vi "OSC_picture.vi"(6 "Falling(T)/Rising(F)":bool, 7 "trig level":dbl format="%#_13g", 8 "error in (no error)":errorcluster, 9 "channels":string="0", 10 "timeout (s) 2":dbl caption="Timeout(s)" format="%.2f", 11 "instrument handle":refnum<k15>) -> (0 "error out":errorcluster, 1 "Waveform Graph":waveform(dbl)[](graph), 2 "the value of the waveform":dbl format="%0.2f", 3 "instrument handle out":refnum<k15>)   [LabVIEW 2013]
uses:
  <instrlib>/niScope/Controls/niScope timestamp type.ctl
  <vilib>/Analysis/baseanly.llb/Mean (DBL).vi
  <vilib>/measure/mamon.llb/Trigger Detection for 1 Channel (obs).vi
  <vilib>/Analysis/NI_AALBase.lvlib
  <vilib>/measure/NI_MAPro.lvlib
panel:
  out "output waveform":waveform(dbl)={"t0"=timestamp(-2.500000000349445e-07 s since 1904-01-01), "dt"=1e-09, "Y"=array[2494 elements]}
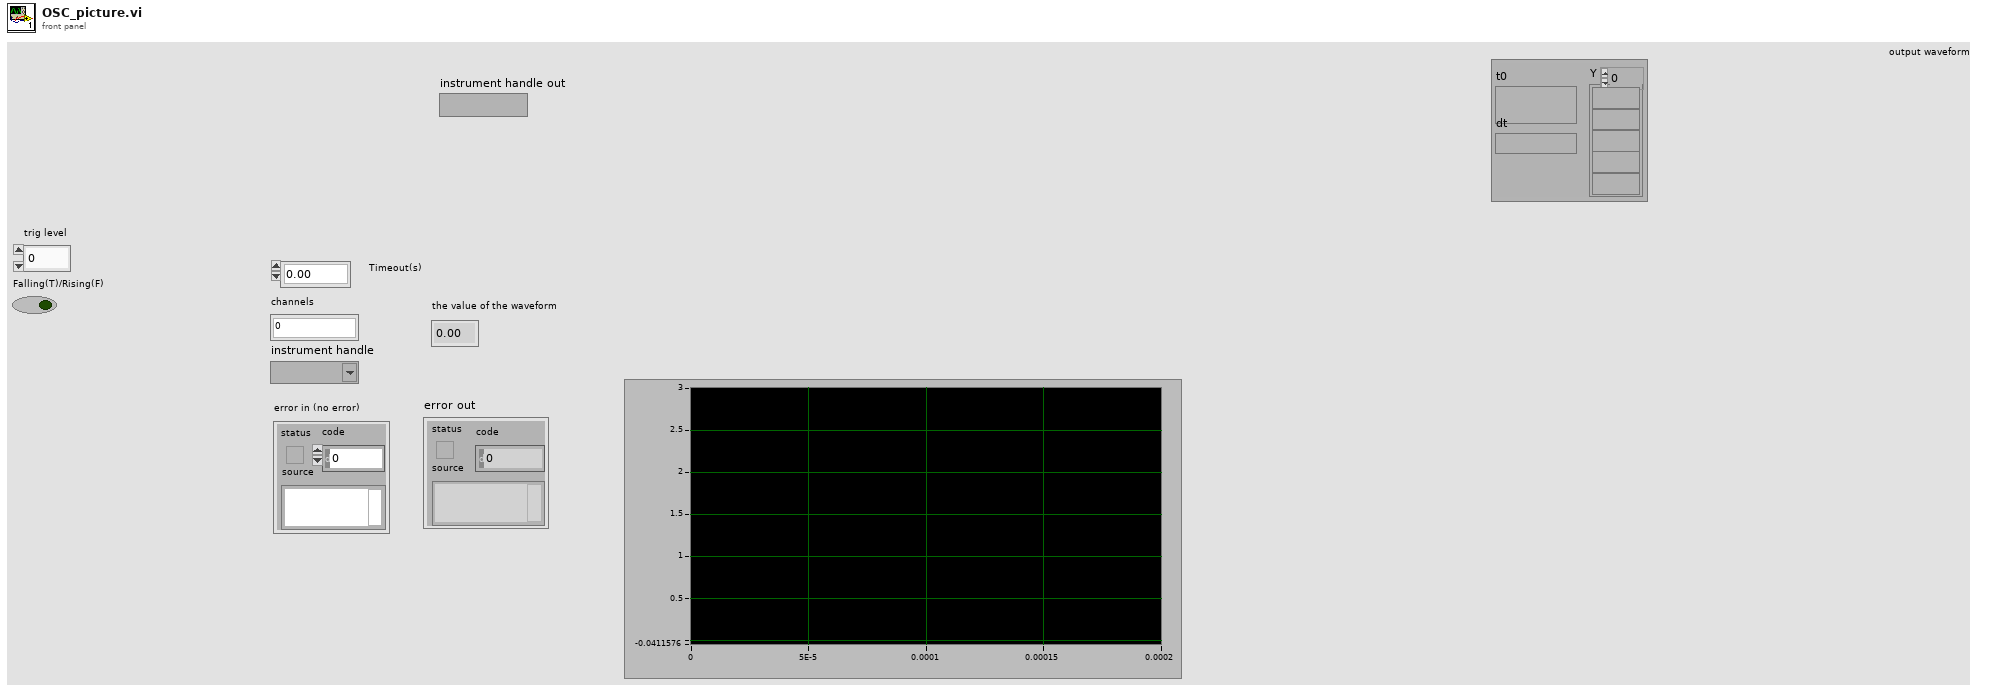
[diagram p1: front panel]
types:
  T1 = typedef "niScope timestamp type.ctl" = i32
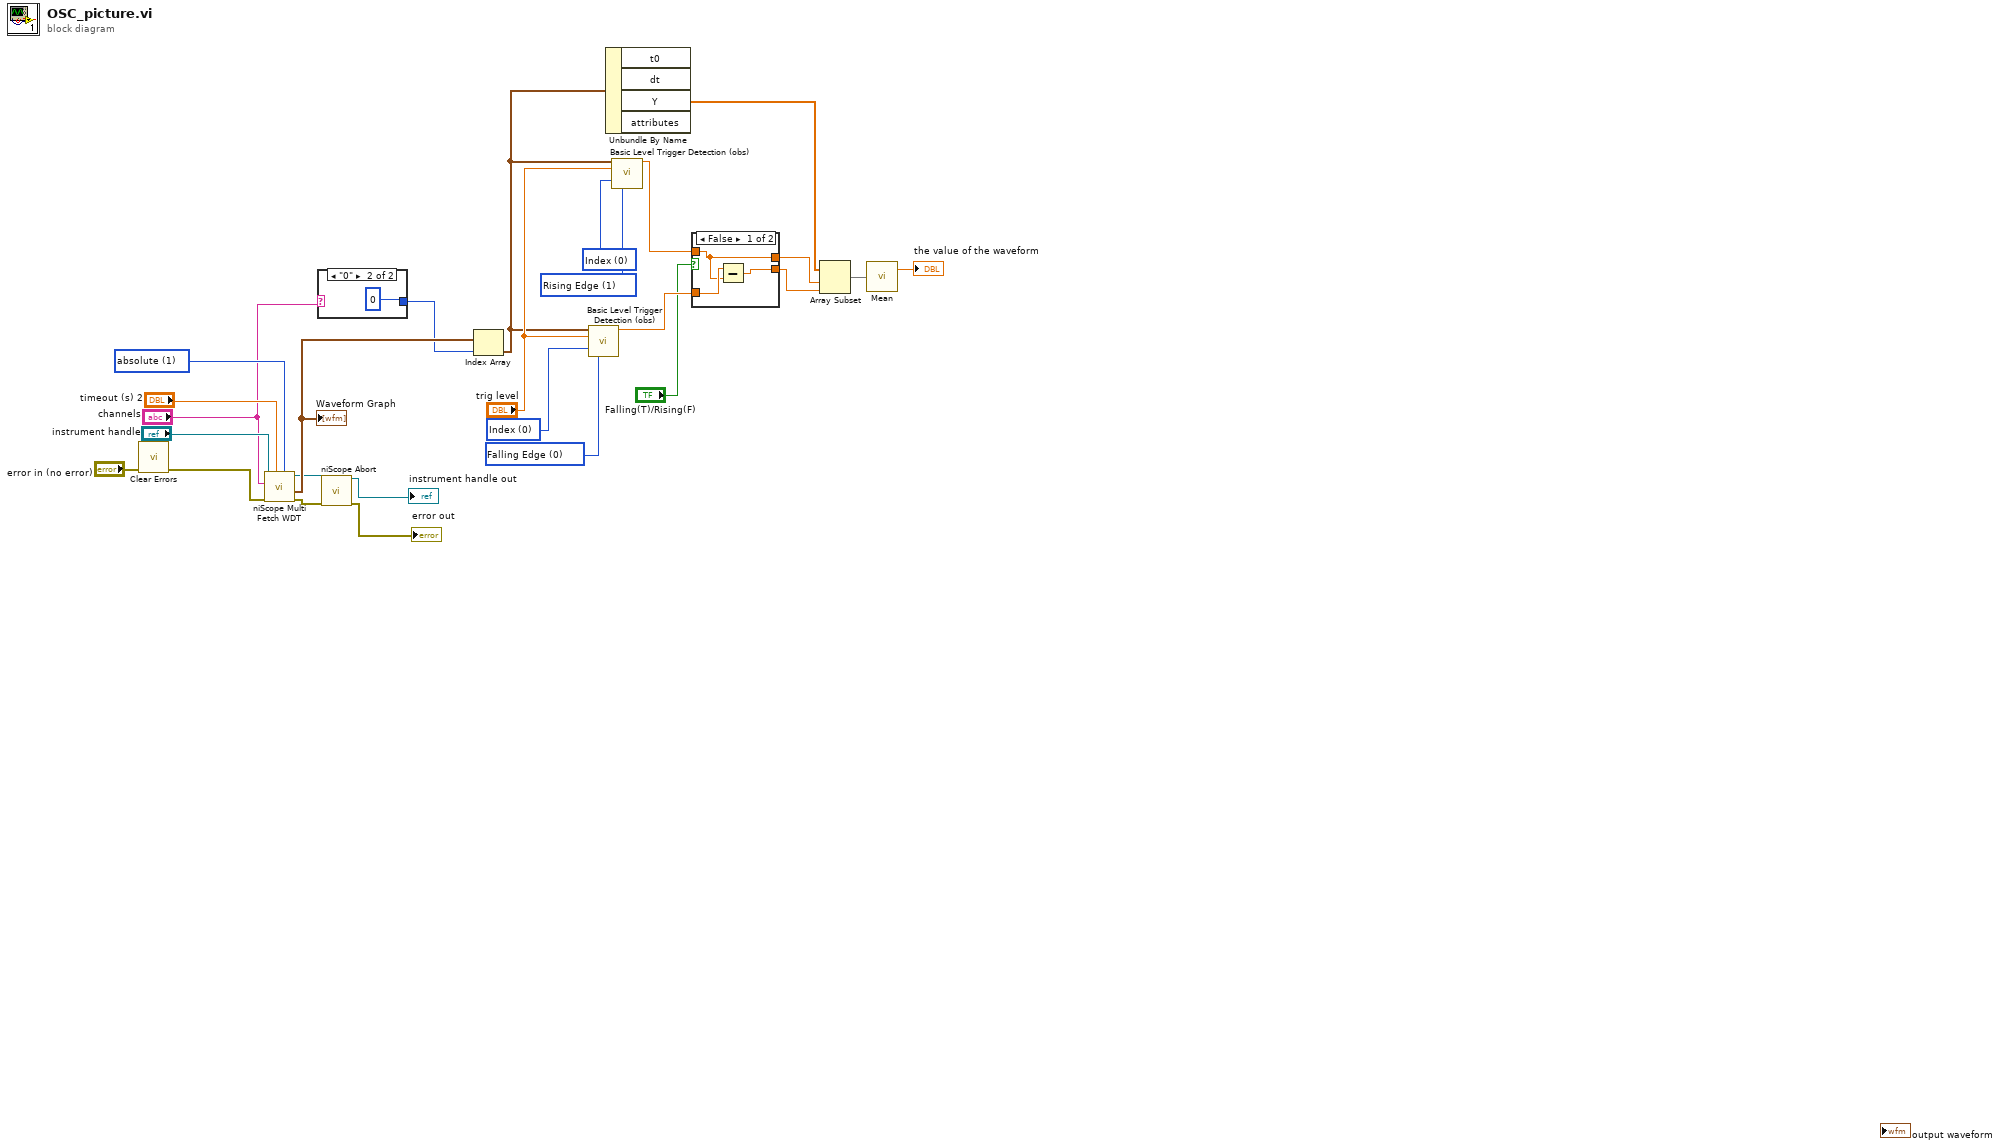
[diagram p0: block diagram]
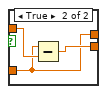
[diagram p2: hidden frame]
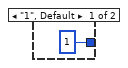
[diagram p3: hidden frame]
diagram:
  w14 = u16 0 items=["Index", "Time"] ("location mode")
  w15 = u16 1 items=["Falling Edge", "Rising Edge"] ("trigger slope")
  w17 = u16 0 items=["Index", "Time"] ("location mode")
  w16 = u16 0 items=["Falling Edge", "Rising Edge"] ("trigger slope")
  w25 = T1 1 items=["relative", "absolute"] ("timestamp Type")
  n1 = call <vilib>:"Clear Errors.vi"("error in (no error)"="error in (no error)") -> ("error out"=w22:errorcluster)  [unwired: 6 in]
  n2 = call "niScope Multi Fetch WDT.vi"("timestamp Type"=w25, "timeout"="timeout (s) 2", "error in"=w22, "channels"="channels", "instrument handle"="instrument handle") -> ("error out"=w3:errorcluster, "wfm"=w21:waveform(dbl)[], "instrument handle out"=w4:refnum<k15>)  [unwired: 3 in, 1 out]
  "Waveform Graph" <- w21
  n3 = case shown="\"0\"" "channels" {
    tunnel: [1 ("index") 0 ("index")] -> w20
    frame "1", Default {
    }
    frame "0" {
    }
  }
  n4 = call <instrlib>:"niScope Abort.vi"("instrument handle"=w4, "error in"=w3) -> ("instrument handle out"=→"instrument handle out":refnum<k15>, "error out"=→"error out":errorcluster)  [unwired: 12 in]
  n5 = Index Array(array=w21, index=w20) -> (element=w10:waveform(dbl))
  n6 = call-poly <vilib>:"Basic Level Trigger Detection (obs).vi"("signal in"=w10, "level"="trig level", "location mode"=w17, "trigger slope"=w16) -> ("trigger location"=w12:dbl)  [unwired: 9 in, 2 out]
  n7 = Unbundle By Name(w10) -> ("Y"=w9:dbl[])  [unwired: 3 out]
  n8 = call-poly <vilib>:"Basic Level Trigger Detection (obs).vi"("signal in"=w10, "level"="trig level", "location mode"=w14, "trigger slope"=w15) -> ("trigger location"=w11:dbl)  [unwired: 9 in, 2 out]
  n9 = case shown="False" "Falling(T)/Rising(F)" {
    tunnel: w12 -> [w30 w32]
    tunnel: w11 -> [w29 w34]
    tunnel: [w31 w33] -> w8
    tunnel: [w29 w32] -> w7
    frame False {
      n10 = Subtract(x=w30, y=w29) -> (x-y=w31:dbl)
    }
    frame True {
      n11 = Subtract(x=w32, y=w34) -> (x-y=w33:dbl)
    }
  }
  n12 = Array Subset(array=w9, index=w7, length=w8) -> (w6:dbl[])
  n13 = call-poly <vilib>:"Mean.vi"("X"=w6) -> ("mean"=→"the value of the waveform":dbl)  [unwired: 1 out]
